vi "Render.vi"(8 "error in":errorcluster, 10 "Renderer in":refnum<class "Renderer.lvclass">, 11 "Lib":refnum<class "Lib.lvclass">) -> (0 "error out":errorcluster, 3 "Sections out":refnum<class "Section.lvclass">[](array[class]))   [LabVIEW 2021, in "TAF Proj Document Type.lvlib" / "Lib.lvclass"]
uses:
  <vilib>/Wovalab/AntiDoc/Document Type/Add-ons/LabVIEW TAF Project/Lib/Lib.lvclass
  C:/Program Files (x86)/National Instruments/LabVIEW 2021/vi.lib/Wovalab/AntiDoc/Bloc/Bloc.lvclass
  <vilib>/Wovalab/AntiDoc/Renderer/Renderer.lvclass
  <vilib>/Wovalab/AsciiDoc for LabVIEW/Section/Section.lvclass
  <vilib>/Wovalab/AntiDoc/Document Type/Add-ons/LabVIEW TAF Project/Lib/Lib.lvclass/Lib.ctl
  <vilib>/Wovalab/AntiDoc/Bloc/Bloc.lvclass/Bloc.ctl
  <vilib>/Wovalab/AntiDoc/Renderer/Renderer.lvclass/Renderer.ctl
  <vilib>/Wovalab/AsciiDoc for LabVIEW/Table/Table.lvclass/Table.ctl
  <vilib>/Wovalab/AntiDoc/Renderer/Read Image Folder Path.vi
  <vilib>/Wovalab/AntiDoc/Bloc/Read Name.vi
  <vilib>/Wovalab/AsciiDoc for LabVIEW/Paragraph/Paragraph.lvclass
  C:/Program Files (x86)/National Instruments/LabVIEW 2021/vi.lib/Wovalab/AsciiDoc for LabVIEW/Adoc-Bloc/Bloc.lvclass
  <vilib>/Wovalab/AsciiDoc for LabVIEW/Table/Table.lvclass
  <vilib>/Wovalab/AsciiDoc for LabVIEW/Section/Add Bloc (array).vi
  <vilib>/Wovalab/AsciiDoc for LabVIEW/Section/Add Bloc (scalar).vi
  <vilib>/Wovalab/AntiDoc/Document Type/Add-ons/LabVIEW TAF Project/Vi/Vi.lvclass
  <vilib>/Wovalab/AntiDoc/Utilities/Utilities.lvlib
  C:/Program Files (x86)/National Instruments/LabVIEW 2021/vi.lib/Wovalab/AsciiDoc for LabVIEW/Paragraph/Paragraph.lvclass
  C:/Program Files (x86)/National Instruments/LabVIEW 2021/vi.lib/Wovalab/AsciiDoc for LabVIEW/Table/Table.lvclass
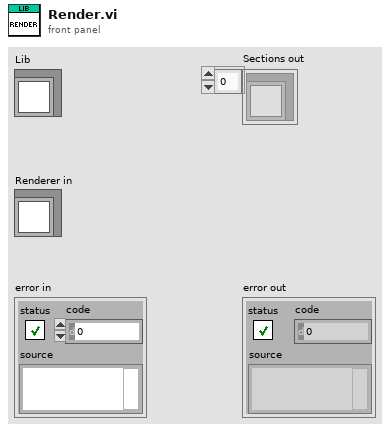
[diagram p1: front panel]
types:
  T1 = typedef "TAF Proj Document Type.lvlib/Lib.lvclass/Nested Lib Info--cluster.ctl" = cluster{"Name":string, "Type":string}
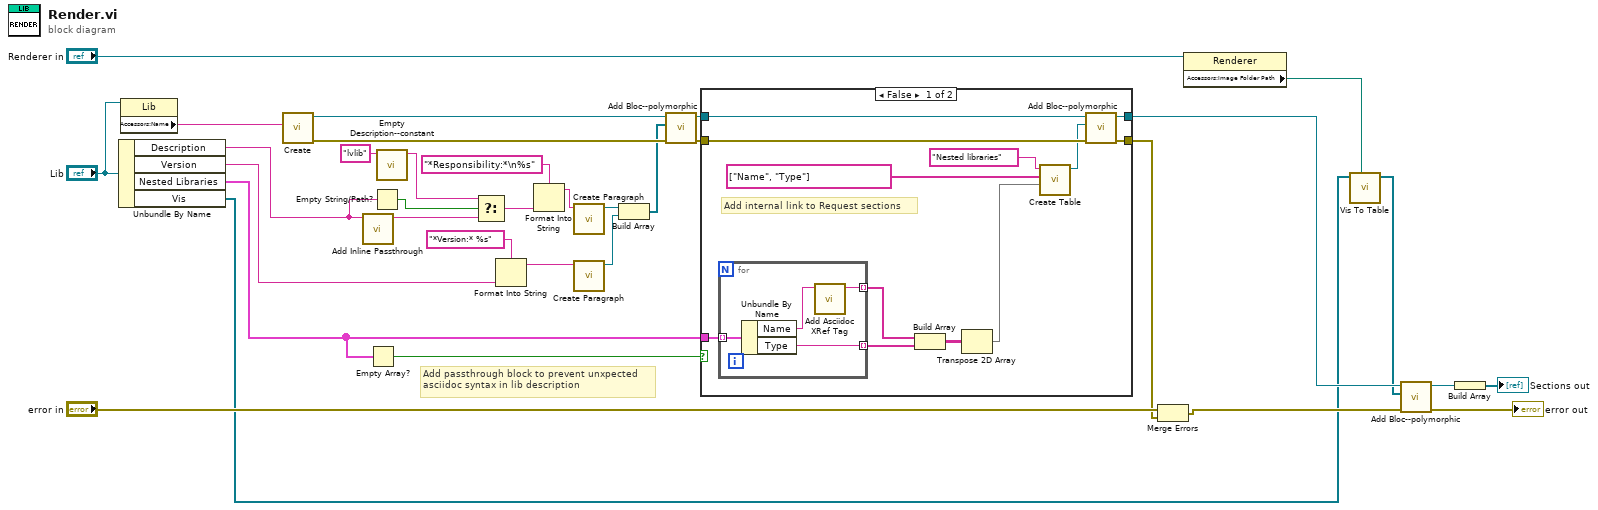
[diagram p0: block diagram]
diagram:
  # "Add passthrough block to prevent unxpected asciidoc syntax in lib description"
  n1 = Unbundle By Name("Lib") -> ("Description"=w2:string, "Version"=w23:string, "Nested Libraries"=w24:T1[], "Vis"=w25:refnum<class "Vi.lvclass">[])
  n2 = property class="Lib"(reference="Lib") -> ("Accessors:Name"=w20:string)  [unwired: 1 in, 2 out]
  n3 = call <vilib>:"Create.vi"("Title"=w20) -> ("error out"=w33:errorcluster, "Section out"=w27:refnum<class "Section.lvclass">)  [unwired: 9 in]
  n4 = call <vilib>:"Add Inline Passthrough.vi"("String in"=w2) -> ("String out"=w1:string)  [unwired: 10 in]
  n5 = Empty Array?(array=w24) -> (empty?=w16:bool)
  n6 = Empty String/Path?(string/path=w2) -> (empty?=w17:bool)
  n7 = call <vilib>:"Empty Description--constant.vi"("Description Source"="lvlib") -> ("Empty Description"=w3:string)  [unwired: 10 in]
  n8 = Select(t=w3, s=w17, f=w1) -> (s? t:f=w11:string)
  n9 = Format Into String(format string="*Version:* %s", w23) -> (resulting string=w8:string)  [unwired: 2 in, 1 out]
  n10 = Format Into String(format string="*Responsibility:*\n%s", w11) -> (resulting string=w10:string)  [unwired: 2 in, 1 out]
  n11 = call <vilib>:"Create Paragraph.vi"("Content"=w10) -> ("Paragraph out"=w18:refnum<class "Paragraph.lvclass">)  [unwired: 9 in, 1 out]
  n12 = call <vilib>:"Create Paragraph.vi"("Content"=w8) -> ("Paragraph out"=w13:refnum<class "Paragraph.lvclass">)  [unwired: 9 in, 1 out]
  n13 = Build Array(w18, w13) -> (w14:refnum<class "Paragraph.lvclass">[])
  n14 = call-poly <vilib>:"Add Bloc--polymorphic.vi"("error in"=w33, "Bloc"=w14, "Section in"=w27) -> ("error out"=w28:errorcluster, "Section out"=w15:refnum<class "Section.lvclass">)  [unwired: 7 in]
  n15 = case shown="False" w16 {
    tunnel: w24 -> [w39 _]
    tunnel: w15 -> [w36 w50]
    tunnel: [w35 w50] -> w26
    tunnel: [w44 w51] -> w29
    tunnel: w28 -> [w45 w51]
    frame False {
      # "Add internal link to Request sections"
      n16 = for {
        tunnel: w39 -> [w49] mode=indexing
        tunnel: [w46] -> w38 mode=indexing
        tunnel: [w48] -> w37 mode=indexing
        n17 = Unbundle By Name(w49) -> ("Name"=w47:string, "Type"=w48:string)
        n18 = call <vilib>:"Add Asciidoc XRef Tag.vi"("String In"=w47) -> ("String out"=w46:string)  [unwired: 10 in]
      }
      n19 = Build Array(w38, w37) -> (w42:string[][])
      n20 = Transpose 2D Array(2D array=w42) -> (transposed array=w43:string[][])
      n21 = call <vilib>:"Create Table.vi"("Content"=w43, "Header"=string[] ["Name", "Type"], "Title"="Nested libraries") -> ("Table out"=w34:refnum<class "Table.lvclass">)  [unwired: 7 in, 1 out]
      n22 = call-poly <vilib>:"Add Bloc--polymorphic.vi"("error in"=w45, "Bloc"=w34, "Section in"=w36) -> ("error out"=w44:errorcluster, "Section out"=w35:refnum<class "Section.lvclass">)  [unwired: 7 in]
    }
    frame True {
    }
  }
  n23 = Merge Errors("error in", w29) -> (w30:errorcluster)
  n24 = property class="Renderer"(reference="Renderer in") -> ("Accessors:Image Folder Path"=w6:path)  [unwired: 1 in, 2 out]
  n25 = call <vilib>:"Vis To Table.vi"("Image Folder Path"=w6, "Vis"=w25) -> ("Table"=w7:refnum<class "Bloc.lvclass">[])  [unwired: 9 in]
  n26 = call-poly <vilib>:"Add Bloc--polymorphic.vi"("error in"=w30, "Bloc"=w7, "Section in"=w26) -> ("error out"=→"error out":errorcluster, "Section out"=w19:refnum<class "Section.lvclass">)  [unwired: 7 in]
  n27 = Build Array(w19) -> (→"Sections out":refnum<class "Section.lvclass">[])
